vi "Init Data.vi"(10 "Data":T1) -> (3 "Msg out":refnum<class "Msg.lvclass">)   [LabVIEW 2020, in "CmdAnalogMultiple.lvlib" / "Msg.lvclass"]
uses:
  Msg.lvclass
  Data.ctl
  CmdAnalog/Data.ctl
  Msg.lvclass/Msg.ctl
  CmdAnalogMultiple.lvlib
  CmdAnalog/CmdAnalog.lvlib
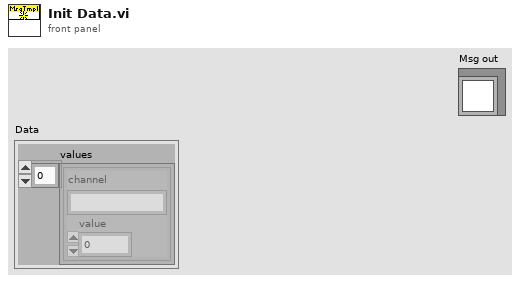
[diagram p1: front panel]
types:
  T1 = typedef "CmdAnalogMultiple.lvlib/Data.ctl" = cluster{"values":T2[]}
  T2 = typedef "CmdAnalog.lvlib/Data.ctl" = cluster{"channel":string, "value":dbl}
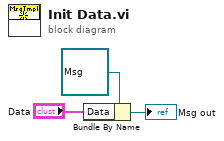
[diagram p0: block diagram]
diagram:
  n1 = Bundle By Name(cluster=refnum<class "Msg.lvclass"> refnum ("Msg out"), "Data"="Data") -> (→"Msg out":refnum<class "Msg.lvclass">)
